vi "Make Barcode Content.vi"(10 "Date":timestamp=timestamp(3743083119.3780074 s since 1904-01-01), 11 "Serial Number":string="12345") -> (3 "Barcode Content":string)   [LabVIEW 2020, in "Barcode Reader Second Iteration.lvlib" / "Barcode Type B Test.lvclass"]
uses:
  Barcode Type B Test.lvclass
  Barcode Type B Test.lvclass/Barcode Type B Test.ctl
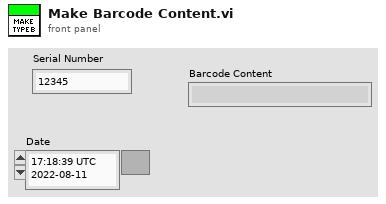
[diagram p1: front panel]
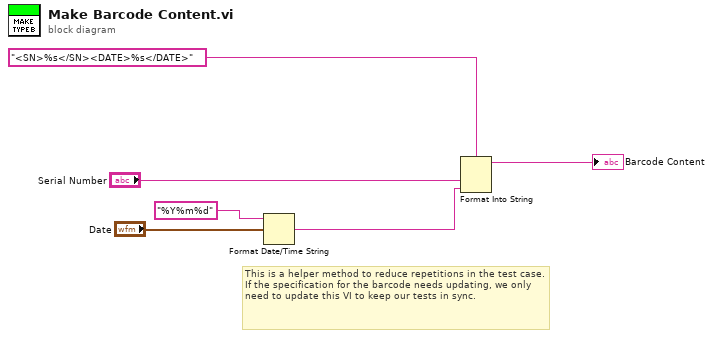
[diagram p0: block diagram]
diagram:
  # "This is a helper method to reduce repetitions in the test case. If the specification for the barcode needs updating, we only need to update this VI to keep our tests in sync."
  n1 = Format Date/Time String(time format string (%c)="%Y%m%d", seconds (now)="Date") -> (date/time string=w1:string)  [unwired: 1 in]
  n2 = Format Into String(format string="<SN>%s</SN><DATE>%s</DATE>" ("Barcode Content"), "Serial Number", w1) -> (resulting string=→"Barcode Content":string)  [unwired: 2 in, 1 out]
